vi "Initialize Status Log.vi"() -> (3 "Status Array":string[](array[string]))   [LabVIEW 2019, in "Dashboard.lvlib"]
uses:
  Dashboard.lvlib
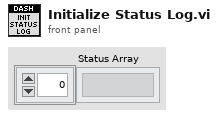
[diagram p1: front panel]
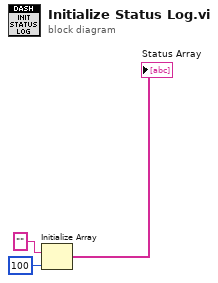
[diagram p0: block diagram]
diagram:
  n1 = Initialize Array("", 100 ("dimension size")) -> (→"Status Array":string[])
